vi "Lorentzian phase test.vi"(3 "output control":T1, 4 "data":variant, 5 "X":dbl[](array[numeric]), 6 "a":dbl[](array[numeric])) -> (0 "error out":errorcluster, 1 "f'(X,a)":dbl[][](array[numeric]), 2 "f(X,a)":dbl[](array[numeric]))   [LabVIEW 2016]
doc: "Sum of three Gaussians, plus DC offset."
uses:
  <vilib>/gmath/NumericalOptimization/LM_output select.ctl
  <vilib>/gmath/NI_Gmath.lvlib
panel:
  out "Waveform Graph":dbl[](graph)
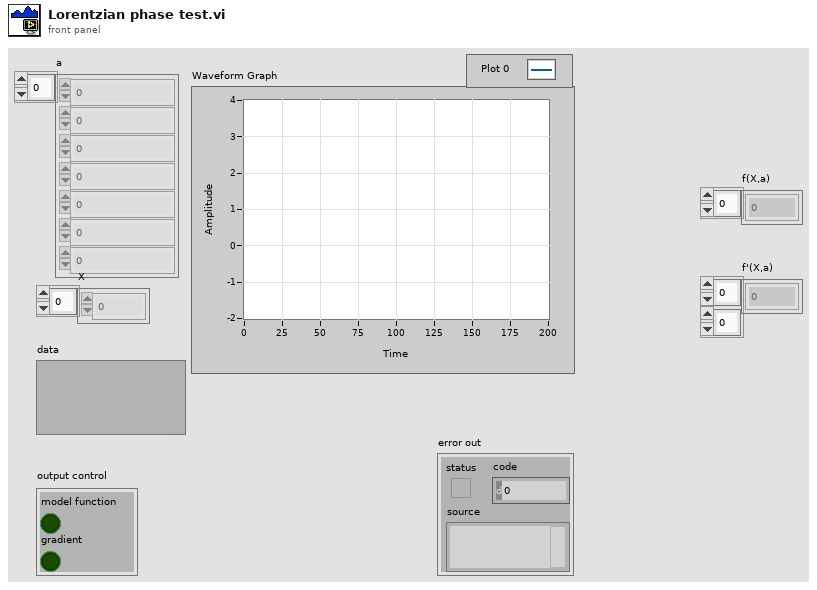
[diagram p1: front panel]
types:
  T1 = typedef "NI_Gmath.lvlib/LM_output select.ctl" = cluster{"model function":bool, "gradient":bool}
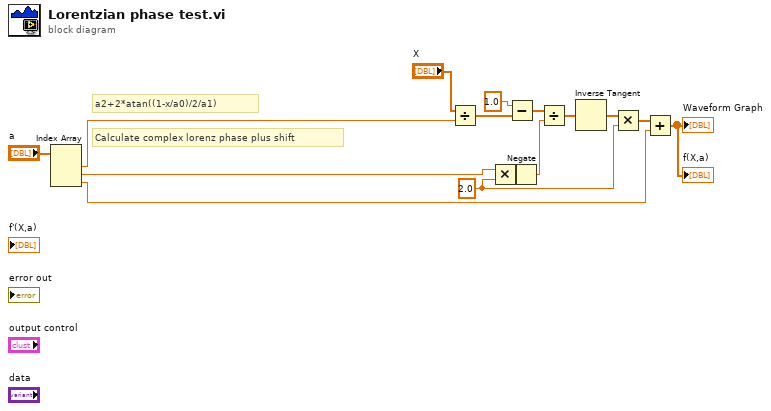
[diagram p0: block diagram]
diagram:
  w6 = 2.0
  # "a2+2*atan((1-x/a0)/2/a1)"
  # "Calculate complex lorenz phase plus shift"
  n1 = Index Array(array="a") -> (element #1=w13:dbl, element #2=w9:dbl, element #3=w3:dbl)  [unwired: 3 in]
  n2 = Divide(x="X", y=w13) -> (x/y=w12:dbl[])
  n3 = Multiply(x=w9, y=w6) -> (x*y=w8:dbl)
  n4 = Subtract(x=1.0, y=w12) -> (x-y=w10:dbl[])
  n5 = Negate(x=w8) -> (-x=w1:dbl)
  n6 = Divide(x=w10, y=w1) -> (x/y=w7:dbl[])
  n7 = Inverse Tangent(1:w7) -> (0:w5:dbl[])
  n8 = Multiply(x=w5, y=w6) -> (x*y=w4:dbl[])
  n9 = Add(x=w4, y=w3) -> (x+y=→"f(X,a)" →"Waveform Graph":dbl[])
